vi "PriorityColoring.vi"(7 "Color Array":u32[](array[colorbox]), 8 "Error In":errorcluster, 10 "Tbl Refnum":refnum<vi>, 11 "SR List In":T1(array[cluster])) -> (0 "Error Out":errorcluster)   [LabVIEW 2017, in "Client.lvlib" / "UI_API.lvlib"]
uses:
  UI_API.lvlib
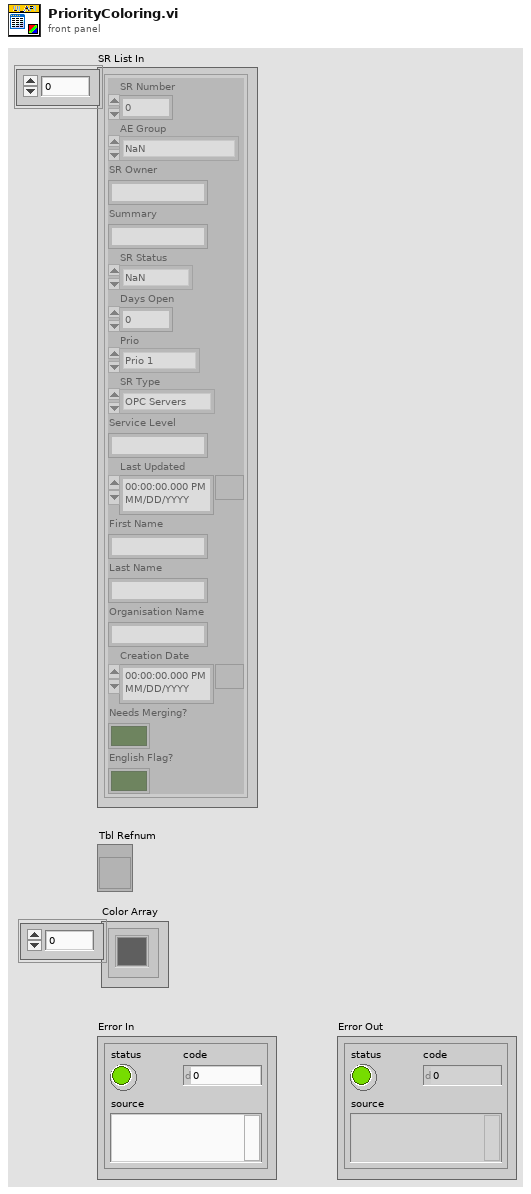
[diagram p1: front panel]
types:
  T1 = cluster{"SR Number":i64, "AE Group":enum32{"NaN", "AE-Germany", "AE-Poland", "AE-Switzerland", "AE-Czech Republic", "AE-Hungary", "AE-Romania", "AE-Slovakia", "AE-Slovenia"}, "SR Owner":string, "Summary":string, "SR Status":enum32{"NaN", "Caller Abandoned", "Created in Error", "Declined to Purchase Support", "Expired", "Forum Resolved AE", "Forum Resolved Customer", "IN WORK", "IN WORK Collab with AES", "IN WORK Collab with PSE", "IN WORK Collab with SE", "IN WORK Escalation", "IN WORK Customer Added Note", "Open", "Potentially Resolved", "POC Resolved", "Resolved", "RMA Waiting on Customer", "RMA Open", "RMA In Progress", "RMA Closed - DOA", "RMA Closed", "RMA Approved for Return", "Project Complete", "Presumed Resolved", "IN WORK Wait on Customer"}, "Days Open":dbl, "Prio":enum16{"Prio 1", "Prio 2", "Prio 3", "Prio 4"}, "SR Type":enum32{"NaN", "ATE Core Configurations (BYOATE)", "Activation", "BioBench", "CAN", "CM C Series", "Calibration", "Consulting Services", "CounterTimer", "DAQExpress", "DASYLab", "DIAdem", "DMM", "DSA HW", "Digital_IO", "FIRST (NIC Only)", "FieldBus", "FieldPoint", "Functional Savety", "GATI", "GPIB", "HMI and Industrial PCs", "HiQ", "HighSpeedDigital_IO", "IMAQ", "IOTech Vibration", "Industrial Communications", "InsightCM", "LV", "LV CD&Sim", "LV Comms", "LV Controls Add-Ons", "LV Embedded", "LV MathScript RT", "LV NXG", "LV NXT", "LVDSC", "LVFPGA", "LVPDA and LV Touch Panel", "LVRT", "LabWindows_CVI", "Lookout", "MATRIXx", "MStudioDotNet", "MStudioVisualBasic", "MStudioVisualC", "Measure (Legacy)", "Motion", "MultifunctionDAQ", "Multimedia Test HW/SW", "Multisim (EWB)", "NI Update Service", "OPC Servers", "Optical (OSI)", "PXI Controllers, Chassis, MXI", "PXI Timing and Sync", "Power Supplies and SMUs", "Powertrain Controls", "RAID", "RF", "RF Software", "RIO", "SC Express", "SCC", "SCXI", "SPEEDY-33 (Hyperception)", "STS", "ScopeDigitizers", "Serial", "Signal Sources", "SignalCondOther", "SignalExpress", "Software Defined Intruments", "Sound and Vibration SW", "Switch Executive", "Switches", "TestStand", "USRP", "Ultiboard (EWB)", "VBench", "VI Logger", "VXI_MXI", "VeriStand", "VisionSW", "VolumeLicenseMgr", "WSN", "Web UI Builder", "myRIO"}, "Service Level":string, "Last Updated":timestamp, "First Name":string, "Last Name":string, "Organisation Name":string, "Creation Date":timestamp, "Needs Merging?":bool, "English Flag?":bool}[]
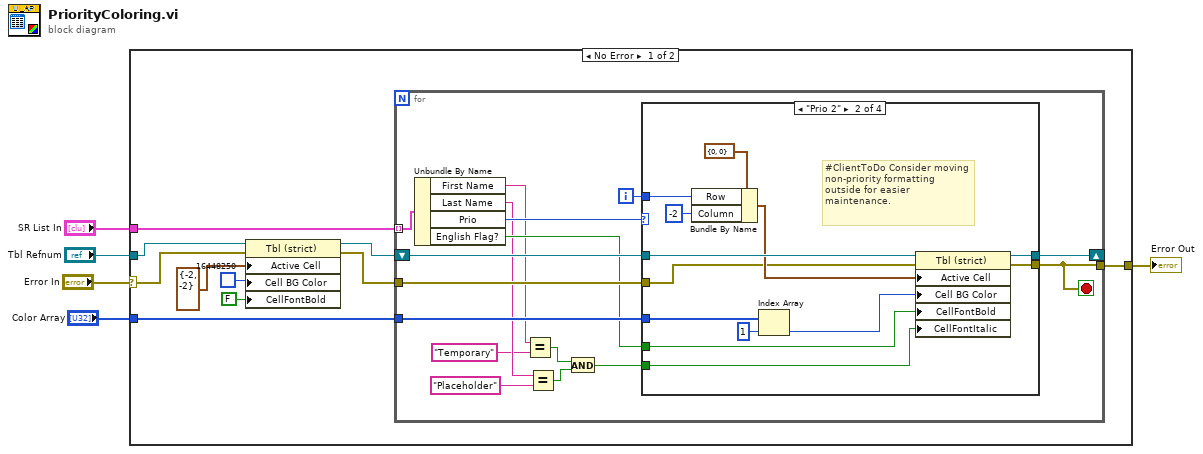
[diagram p0: block diagram]
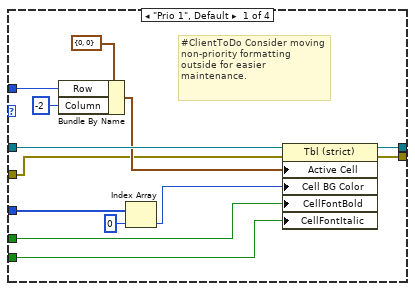
[diagram p2: hidden frame]
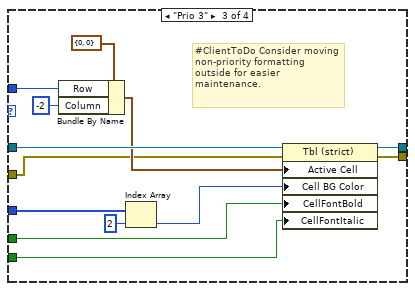
[diagram p3: hidden frame]
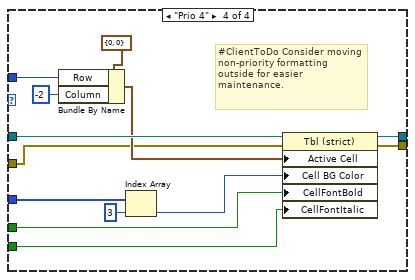
[diagram p4: hidden frame]
diagram:
  n1 = case shown="No Error" "Error In" {
    selector: "Error In" -> [w6 w84]
    tunnel: "SR List In" -> [w9 _]
    tunnel: "Tbl Refnum" -> [w7 _]
    tunnel: "Color Array" -> [w15 _]
    tunnel: [w8 w84] -> w1
    frame No Error {
      n2 = property class="Tbl (strict)"(reference=w7, error in=w6, "Active Cell"=cluster{"Row":i32, "Column":i32} {"Row"=-2, "Column"=-2} ("Active Cell:Active Cell"), "Cell BG Color"=u32 16448250, "CellFontBold"=FALSE) -> (reference out=w11:refnum<vi>, error out=w10:errorcluster)
      n3 = for {
        tunnel: w9 -> [w31] mode=indexing
        tunnel: w15 -> [w29]
        shift-right: [w27] -> _
        shift-left: w11 -> [w30]
        tunnel: w10 -> [w26]
        tunnel: [w25] -> w8
        i -> [w28]
        stop <- w25 stop-if-true
        n4 = Unbundle By Name(w31) -> ("First Name"=w19:string, "Last Name"=w18:string, "Prio"=w24:enum16{"Prio 1", "Prio 2", "Prio 3", "Prio 4"}, "English Flag?"=w23:bool)
        n5 = Equal?(x=w19, y="Temporary") -> (x = y?=w22:bool)
        n6 = Equal?(x=w18, y="Placeholder") -> (x = y?=w21:bool)
        n7 = And(x=w22, y=w21) -> (x .and. y?=w20:bool)
        n8 = case shown="\"Prio 2\"" w24 {
          tunnel: w30 -> [w44 w57 w70 w83]
          tunnel: w29 -> [w39 w52 w65 w78]
          tunnel: w28 -> [w42 w55 w68 w81]
          tunnel: [w36 w49 w62 w75] -> w27
          tunnel: w26 -> [w35 w48 w61 w74]
          tunnel: [w34 w47 w60 w73] -> w25
          tunnel: w23 -> [w33 w46 w59 w72]
          tunnel: w20 -> [w32 w45 w58 w71]
          frame "Prio 1", Default {
            # "#ClientToDo Consider moving non-priority formatting outside for easier maintenance."
            n9 = Bundle By Name(cluster=cluster{"Row":i32, "Column":i32} {"Row"=0, "Column"=0} ("Active Cell:Active Cell"), "Row"=w42, "Column"=-2) -> (w40:cluster{"Row":i32, "Column":i32})
            n10 = Index Array(array=w39, index=0) -> (element=w38:u32)
            n11 = property class="Tbl (strict)"(reference=w44, error in=w35, "Active Cell"=w40, "Cell BG Color"=w38, "CellFontBold"=w33, "CellFontItalic"=w32) -> (reference out=w36:refnum<vi>, error out=w34:errorcluster)
          }
          frame "Prio 2" {
            # "#ClientToDo Consider moving non-priority formatting outside for easier maintenance."
            n12 = Bundle By Name(cluster=cluster{"Row":i32, "Column":i32} {"Row"=0, "Column"=0} ("Active Cell:Active Cell"), "Row"=w55, "Column"=-2) -> (w53:cluster{"Row":i32, "Column":i32})
            n13 = Index Array(array=w52, index=1) -> (element=w51:u32)
            n14 = property class="Tbl (strict)"(reference=w57, error in=w48, "Active Cell"=w53, "Cell BG Color"=w51, "CellFontBold"=w46, "CellFontItalic"=w45) -> (reference out=w49:refnum<vi>, error out=w47:errorcluster)
          }
          frame "Prio 3" {
            # "#ClientToDo Consider moving non-priority formatting outside for easier maintenance."
            n15 = Bundle By Name(cluster=cluster{"Row":i32, "Column":i32} {"Row"=0, "Column"=0} ("Active Cell:Active Cell"), "Row"=w68, "Column"=-2) -> (w66:cluster{"Row":i32, "Column":i32})
            n16 = Index Array(array=w65, index=2) -> (element=w64:u32)
            n17 = property class="Tbl (strict)"(reference=w70, error in=w61, "Active Cell"=w66, "Cell BG Color"=w64, "CellFontBold"=w59, "CellFontItalic"=w58) -> (reference out=w62:refnum<vi>, error out=w60:errorcluster)
          }
          frame "Prio 4" {
            # "#ClientToDo Consider moving non-priority formatting outside for easier maintenance."
            n18 = Bundle By Name(cluster=cluster{"Row":i32, "Column":i32} {"Row"=0, "Column"=0} ("Active Cell:Active Cell"), "Row"=w81, "Column"=-2) -> (w79:cluster{"Row":i32, "Column":i32})
            n19 = Index Array(array=w78, index=3) -> (element=w77:u32)
            n20 = property class="Tbl (strict)"(reference=w83, error in=w74, "Active Cell"=w79, "Cell BG Color"=w77, "CellFontBold"=w72, "CellFontItalic"=w71) -> (reference out=w75:refnum<vi>, error out=w73:errorcluster)
          }
        }
      }
    }
    frame Error {
    }
  }
  "Error Out" <- w1
